vi "Multirecord Acquisition (FPGA).vi"() -> ()   [LabVIEW 2021]
doc: "Use this VI as a template for the reconfigurable oscilloscope acquisition design. The block diagram is divided into three main loops.\n\nRegister Bus: This loop initializes the registers that are needed to support the configuration of the device. The FIFO bus, on the left, allows all the other design libraries to communicate with one another. This loop is very important to support the proper behavior of the instrument design library components.\n\nAcquisition: Acquires data from the I/O channels and writes the data into the record memory using the <B>Write</B> VI of the Multirecord Acquisition instrument design library. This VI also evaluates the various acquisition triggers and decides whether to acquire each data value in record memory. The host level VI (Fetch Record.vi) can read acquired records from the DRAM. The data is stored in 2 DRAM banks, each with 768 MB of storage.\n\nFetch: The recorded data is retrieved when the <B>Fetch Single Record</B> VI is run from the host VI. The <B>Write to Fetch DMA FIFO</B> VI writes data to the acq.fetch fifo 0 to transmit record data form the FPGA to the record fetch VIs on the host. This DMA FIFO must have a predefined name based on the instance parameter. By default, it is 0 (since the associated terminal on the <B>Create Resources DRAM Write Read</B> VI is unwired), so the connected FIFO is named acq.fetch fifo 0."
uses:
  Trigger/SubVIs/Types/Trigger Type.ctl
  <instrlib>/_niInstr/Data Trigger/v1/Shared/Public/Level Configuration FXP(+-,18,1).ctl
  <instrlib>/_niInstr/Data Trigger/v1/Shared/Public/Level Configuration Trigger When.ctl
  <instrlib>/_niInstr/Data Trigger/v1/Shared/Public/Edge Configuration FXP(+-,18,1).ctl
  <instrlib>/_niInstr/Data Trigger/v1/Shared/Public/Edge Configuration Trigger Slope.ctl
  FPGA Interface Typedefinitions/Trigger Combination Type.ctl
  <vilib>/Platform/TimedLoop/XDataNode/timing_clust.ctl
  <vilib>/Platform/TimedLoop/XDataNode/nitl_modes.ctl
  <vilib>/Platform/TimedLoop/XDataNode/wakeup.ctl
  <instrlib>/_niInstr/FIFO Register Bus/v1/FPGA/niInstr FIFO Register Bus v1 FPGA.lvclass
  C:/Program Files (x86)/National Instruments/LabVIEW 2021/instr.lib/_niInstr/Instruction Framework/v1/FPGA/Interfaces/Instruction Producer/Instruction Producer.lvclass
  <instrlib>/_niInstr/Multirecord Acquisition/Common/v1/FPGA/niInstr Multirecord Acquisition Common v1 FPGA.lvclass
  C:/Program Files (x86)/National Instruments/LabVIEW 2021/instr.lib/_niInstr/Multirecord Acquisition/Interface/v1/FPGA/niInstr Multirecord Acquisition v1 FPGA.lvclass
  <vilib>/rvi/Emulation/niFpgaSctlEmulationGetInTimedLoop.vi
  <vilib>/rvi/Emulation/niFpgaEmulationReportErrorSimple.vi
  <vilib>/rvi/Emulation/niFpgaGetClockAttributes.vi
  <vilib>/rvi/Emulation/niFpgaCriticalErrorInLSC.vi
  <instrlib>/_niInstr/Multirecord Acquisition/Common/v1/FPGA/Private/Create Fetch DMA FIFO Resources U8x32.vi
  <instrlib>/_niInstr/Multirecord Acquisition/Common/v1/FPGA/Private/Create Resources DRAM U384x2 U768 Write Read.vi
  <vilib>/rvi/eio/common/nirviEmuTemplateMethod_errors.vi
  <instrlib>/HSAI-RIO/Config/Group A/v1/FPGA/Digital Correction/Validate 8 Channel Data.vi
  <instrlib>/HSAI-RIO/Config/Group A/v1/FPGA/Digital Correction/Digital Correction (8 Ch).vi
  <instrlib>/HSAI-RIO/Config/Group A/v1/FPGA/Digital Correction/FIR Filter (8 Ch).vi
  DSP/SubVIs/Integer decimationx8ch.vi
  Data Type Conversion/SubVIs/Remove Overflow FXP(+-,18,1)x8ch.vi
  <instrlib>/_niInstr/Channel/v1/FPGA/Private/Select/Select FXP(+-,18,1,)xNspcx8ch.vi
  Trigger/Trigger FXP(+,-,18,1).vi
  Data Type Conversion/SubVIs/Data Type Conversion FXP(+-,18,1) to I16x8ch.vi
  <instrlib>/_niInstr/Channel/v1/FPGA/Private/Select and Interleave/Select And Interleave I16xNspcx8ch.vi
  <instrlib>/_niInstr/Multirecord Acquisition/Interface/v1/FPGA/Private/Write I16 Wrapper.vi
  <vilib>/Platform/TimedLoop/XDataNode/XDataNode.xnode
  <vilib>/eio/EIONode/EIONode.xnode
  <instrlib>/_niInstr/Instruction Framework/v1/FPGA/Top Level Bus/Register Configuration/Register Configuration.lvclass
  <vilib>/Platform/TimedLoop/XDataNode/XDNodeRunTimeDep.lvlib
  <instrlib>/_niInstr/Multirecord Acquisition/Interface/v1/FPGA/niInstr Multirecord Acquisition v1 FPGA.lvclass
  <vilib>/rvi/LocalResourceManager/LocalResourceManager.xnode
  <vilib>/rvi/eio/common/nirviEmuReportErrorAndStop.vi
  <vilib>/rvi/DataTransferAndStorage/Container/Common/niFpgaContainerGetUniqueNameForEmu.vi
  <vilib>/rvi/DataTransferAndStorage/Container/Common/niFpgaContainerSetEmuInfo.vi
  <instrlib>/_niInstr/Channel/v1/FPGA/niInstr Channel v1 FPGA.lvlib
  <instrlib>/_niInstr/Basic Elements/v1/FPGA/niInstr Basic Elements v1 FPGA.lvlib
  <instrlib>/HSAI-RIO/Config/Group A/v1/FPGA/Digital Correction/Digital Correction.lvclass
  <instrlib>/HSAI-RIO/Config/Group A/v1/FPGA/Config Registers/Config Registers.lvclass
  <instrlib>/_niInstr/Data Trigger/v1/Shared/niInstr Data Trigger v1 Shared.lvlib
  Emulation/SubVIs/2 Element Generate Sine Cos Data FXP(+,-,14,1).vi
  <instrlib>/_niInstr/Multirecord Acquisition/Common/v1/FPGA/Private/Create Resources DRAM U384.vi
  <instrlib>/_niInstr/Multirecord Acquisition/Common/v1/FPGA/Private/Create Resources BRAM U384.vi
  <instrlib>/_niInstr/Multirecord Acquisition/Common/v1/FPGA/Private/Create Resources BRAM U768.vi
  C:/Program Files (x86)/National Instruments/LabVIEW 2021/instr.lib/_niInstr/Multirecord Acquisition/Common/v1/FPGA/niInstr Multirecord Acquisition Common v1 FPGA.lvclass
  FPGA Interface Typedefinitions/FPGA Interface Typedefinitions.lvlib
panel:
  in  "trigger.combination type":T1
  in  "trigger.rearm delay":u16=2
  in  "start trigger":bool=TRUE
  in  "trigger.type B":T2
  in  "reset":bool
  in  "trigger.edge B":T3
  in  "trigger.level B":T5
  in  "trigger.edge A":T3
  in  "trigger.level A":T5
  in  "trigger.type A":T2
  in  "trigger.channel A":u8
  in  "trigger.channel B":u8
  out "fifo reg bus data 0":u64
  out "fifo reg bus status 0":u32
  in  "fifo reg bus ctrl 0":u32
  out "overflow":bool
  in  "dsp.decimation factor":u16
  out "overload":bool
  in  "channel.enable mask":u16=65535 format="%.0b"
  in  "channel.number of channels":u8=8
  # "Register Bus Controls"
  # "FPGA"
  # "Acquisition Loop Controls"
  # "DSP"
  # "Trigger"
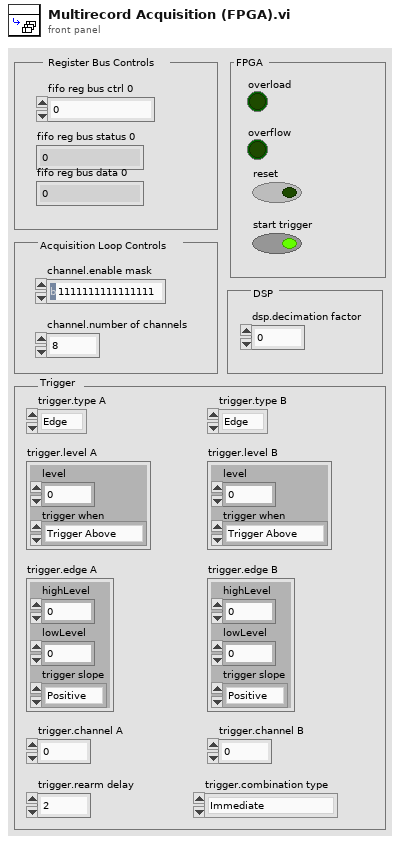
[diagram p1: front panel]
types:
  T1 = typedef "FPGA Interface Typedefinitions.lvlib/Trigger Combination Type.ctl" = enum16{"Immediate", "A", "B", "OR", "AND", "A THEN B", "B THEN A", "High Resolution"}
  T2 = typedef "Trigger Type.ctl" = enum16{"Edge", "Level", "Custom"}
  T3 = typedef "niInstr Data Trigger v1 Shared.lvlib/Edge Configuration FXP(+-,18,1).ctl" = cluster{"highLevel":fxp<+/-,18,1>, "lowLevel":fxp<+/-,18,1>, "trigger slope":T4}
  T4 = typedef "niInstr Data Trigger v1 Shared.lvlib/Edge Configuration Trigger Slope.ctl" = enum8{"Positive", "Negative"}
  T5 = typedef "niInstr Data Trigger v1 Shared.lvlib/Level Configuration FXP(+-,18,1).ctl" = cluster{"level":fxp<+/-,18,1>, "trigger when":T6}
  T6 = typedef "niInstr Data Trigger v1 Shared.lvlib/Level Configuration Trigger When.ctl" = enum8{"Trigger Above", "Trigger Below"}
  T7 = cluster{"memory 1":refnum<k21>, "memory 2":refnum<k21>}
  T8 = typedef "XDNodeRunTimeDep.lvlib/timing_clust.ctl" = cluster{"Expected End [f-1]":u64, "Actual End [f-1]":u64, "Finished Late? [f-1]":bool, "Expected End [i-1]":u64, "Actual End [i-1]":u64, "Finished Late? [i-1]":bool, "Expected Start [i]":u64, "Actual Start [i]":u64, "Expected Start [f]":u64, "Actual Start [f]":u64, "Source Name":string, "Structure Name":string, "Period":i64, "Deadline":i64, "Offset":i64, "Start":i64, "Priority":i32, "Timeout":i32, "Mode":T9, "Wakeup Reason":T10, "Error":errorcluster, "Source Type":string, "Secondary Source Type":string, "Global End Time":u64, "Global Start Time":u64, "Frame Duration":u64, "Iteration Duration":u64, "Assigned CPU":i32, "I/O Scan Engine Mode":u32}
  T9 = typedef "XDNodeRunTimeDep.lvlib/nitl_modes.ctl" = enum32{"No Change", "Process missed periods, maintain original phase", "Discard missed periods, maintain original phase", "Process missed periods, ignore original phase", "Discard missed periods, ignore original phase"}
  T10 = typedef "XDNodeRunTimeDep.lvlib/wakeup.ctl" = enum32{"Normal", "Aborted", "Asynchronous wakeup", "Timing source error", "Timed loop error", "Timeout"}
  T11 = cluster{"Channel 0":fxp<+/-,14,1>[], "Channel 1":fxp<+/-,14,1>[], "Channel 2":fxp<+/-,14,1>[], "Channel 3":fxp<+/-,14,1>[], "Channel 4":fxp<+/-,14,1>[], "Channel 5":fxp<+/-,14,1>[], "Channel 6":fxp<+/-,14,1>[], "Channel 7":fxp<+/-,14,1>[]}
  T12 = cluster{"Channel 0":fxp<+/-,18,1>[], "Channel 1":fxp<+/-,18,1>[], "Channel 2":fxp<+/-,18,1>[], "Channel 3":fxp<+/-,18,1>[], "Channel 4":fxp<+/-,18,1>[], "Channel 5":fxp<+/-,18,1>[], "Channel 6":fxp<+/-,18,1>[], "Channel 7":fxp<+/-,18,1>[]}
  T13 = cluster{"channel 0":fxp<+/-,18,1>[], "channel 1":fxp<+/-,18,1>[], "channel 2":fxp<+/-,18,1>[], "channel 3":fxp<+/-,18,1>[], "channel 4":fxp<+/-,18,1>[], "channel 5":fxp<+/-,18,1>[], "channel 6":fxp<+/-,18,1>[], "channel 7":fxp<+/-,18,1>[]}
  T14 = cluster{"channel 0":i16[], "channel 1":i16[], "channel 2":i16[], "channel 3":i16[], "channel 4":i16[], "channel 5":i16[], "channel 6":i16[], "channel 7":i16[]}
  T15 = typedef "niInstr Multirecord Acquisition v1 FPGA.lvclass/Timestamp.ctl" = cluster{"timestamp":u64, "valid":bool}
  T16 = typedef "niInstr Types v1 Shared.lvlib/Input Triggers.ctl" = cluster{"start":bool, "advance":bool, "reference":bool, "start trigger index":u16, "advance trigger index":u16, "reference trigger index":u16, "reference trigger correction cycle count":u32}
  T17 = typedef "niInstr Types v1 Shared.lvlib/Sample Format.ctl" = cluster{"bits per channel":u16, "samples per clock":u16, "channels":u8}
  T18 = typedef "niInstr Multirecord Acquisition v1 FPGA.lvclass/Events.ctl" = cluster{"ready for start":bool, "ready for advance":bool, "ready for reference":bool, "end of record":bool, "done":bool, "start trigger":bool, "advance trigger":bool, "reference trigger":bool, "start trigger index":u16, "advance trigger index":u16, "reference trigger index":u16}
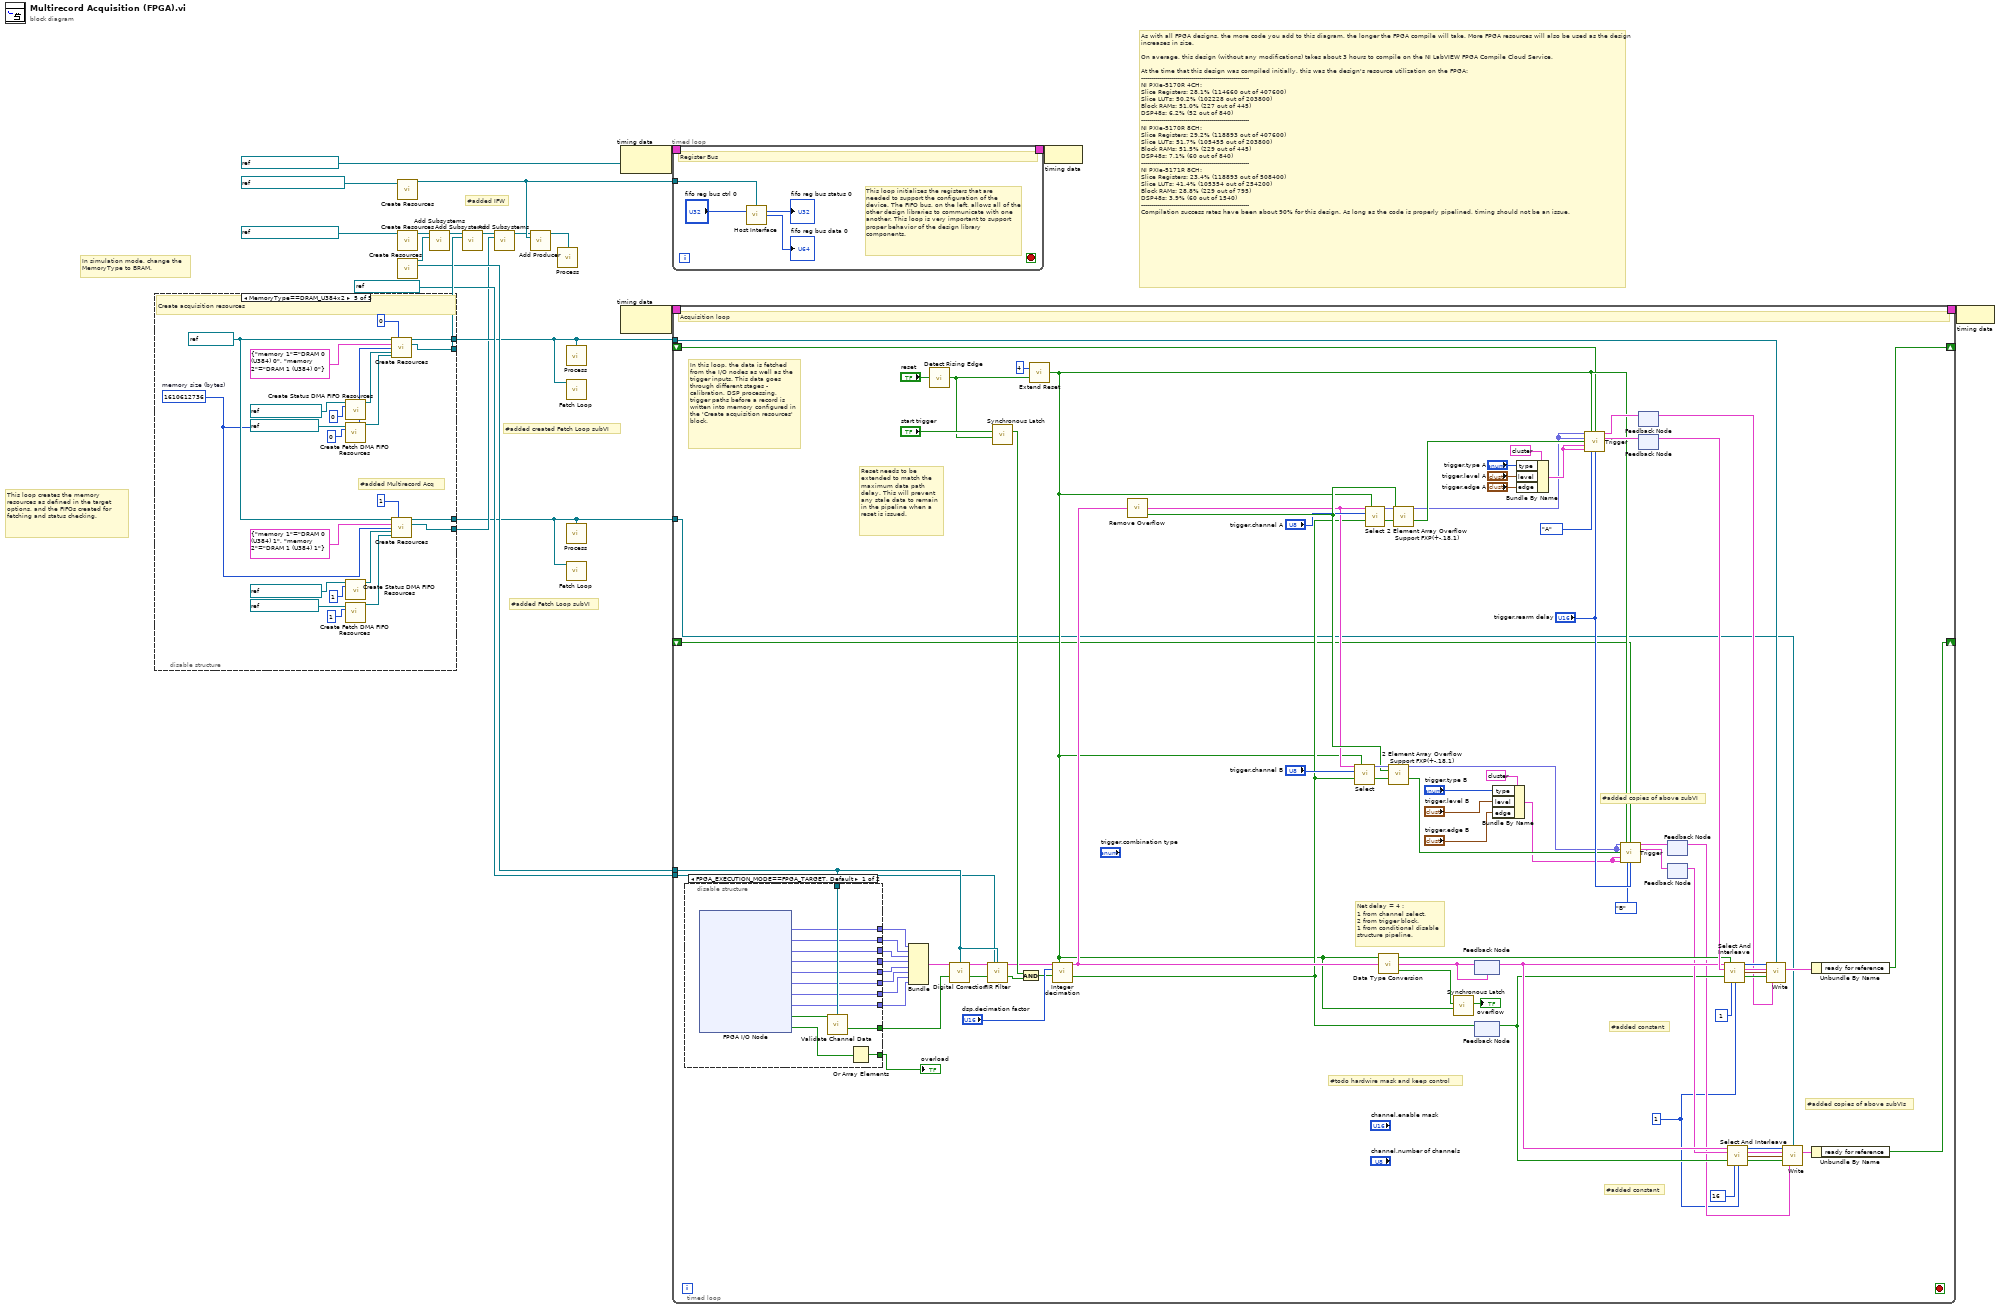
[diagram p0: block diagram]
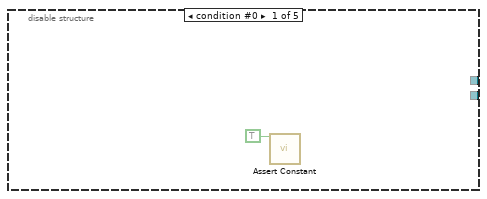
[diagram p2: hidden frame]
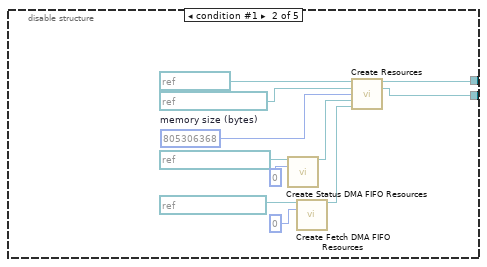
[diagram p3: hidden frame]
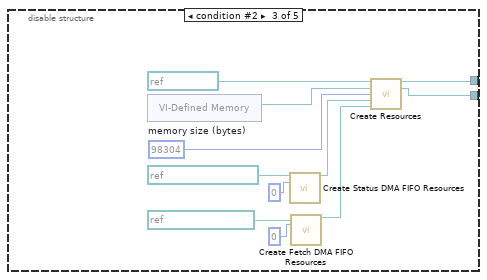
[diagram p4: hidden frame]
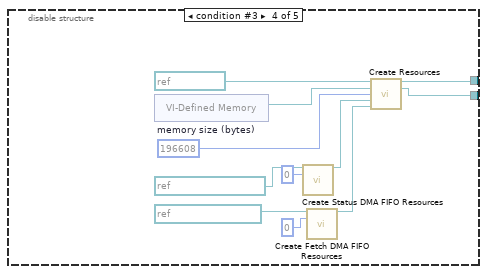
[diagram p5: hidden frame]
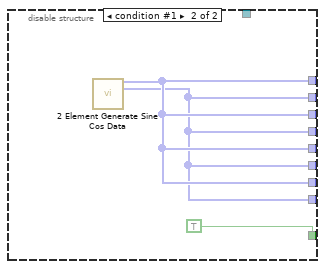
[diagram p6: hidden frame]
diagram:
  # "#added created Fetch Loop subVI"
  # "#added Fetch Loop subVI"
  # "#added IFW"
  # "In simulation mode, change the MemoryType to BRAM."
  # "This loop creates the memory resources as defined in the target options, and the FIFOs created for fetching and status checking."
  # "As with all FPGA designs, the more code you add to this diagram, the longer the FPGA compile will take. More FPGA resources will also be used as the design increases in size.\n\nOn average, this design (without any modifications) takes about 3 hours to compile on the NI LabVIEW FPGA Compile Cloud Service. \n\nAt the time that this design was compiled initially, this was the design's resource utilization on the FPGA:\n------------------------------------------------------\nNI PXIe-5170R 4CH:\nSlice Registers: 28.1% (114660 out of 407600)\nSlice LUTs: 50.2% (102228 out of 203800)\nBlock RAMs: 51.0% (227 out of 445)\nDSP48s: 6.2% (52 out of 840)\n------------------------------------------------------\nNI PXIe-5170R 8CH:\nSlice Registers: 29.2% (118893 out of 407600)\nSlice LUTs: 51.7% (105455 out of 203800)\nBlock RAMs: 51.5% (229 out of 445)\nDSP48s: 7.1% (60 out of 840)\n------------------------------------------------------\nNI PXIe-5171R 8CH:\nSlice Registers: 23.4% (118893 out of 508400)\nSlice LUTs: 41.4% (105354 out of 254200)\nBlock RAMs: 28.8% (229 out of 795)\nDSP48s: 3.9% (60 out of 1540)\n------------------------------------------------------\nCompilation success rates have been about 90% for this design. As long as the code is properly pipelined, timing should not be an issue."
  n1 = disable-structure shown="MemoryType==DRAM_U384x2" {
    disable-tunnel: [_ w30 w41 w52 w76] -> w3
    disable-tunnel: [_ w27 w37 w48 w73] -> w10
    disable-tunnel: [_ _ _ _ w56] -> w1
    disable-tunnel: [_ _ _ _ w55] -> w2
    frame condition #0 {
      n2 = call <instrlib>:"Assert Constant.vi"("constant terminal"=TRUE) -> ()  [unwired: 15 in]
    }
    frame condition #1 {
      w31 = u64 805306368  # memory size (bytes)
      n3 = call <instrlib>:"Create Status DMA FIFO Resources.vi"("status dma fifo in"=refnum<k21> "acq.status fifo 0" ("status dma fifo"), "fifo instance"=u8 0) -> ("status dma fifo out"=w22:refnum<class "niInstr Status FIFO v1 FPGA.lvclass">)  [unwired: 13 in]
      n4 = call-poly <instrlib>:"Create Fetch DMA FIFO Resources.vi"("fetch dma fifo in"=refnum<k21> "acq.fetch fifo 0", "fifo instance"=u8 0) -> ("fetch dma fifo out"=w28:refnum<class "niInstr Fetch FIFO v1 FPGA.lvclass">)  [unwired: 13 in]
      n5 = call-poly <instrlib>:"Create Resources.vi"("memory clock"=refnum<k21> "160MHz" ("process clock"), "memory"=refnum<k21> "DRAM 0 (U384)" ("dram"), "memory size (bytes)"=w31, "status dma fifo resources"=w22, "fetch dma fifo resources"=w28) -> ("acquisition resources"=w30:refnum<class "niInstr Multirecord Acquisition Common v1 FPGA.lvclass">, "acquisition subsystem"=w27:refnum<class "Address Space Collection.lvclass">)  [unwired: 9 in]
    }
    frame condition #2 {
      w42 = u64 98304  # memory size (bytes)
      n6 = xnode "VI-Defined Memory"() -> ("Memory Out"=w43:refnum<k21>)
      n7 = call <instrlib>:"Create Status DMA FIFO Resources.vi"("status dma fifo in"=refnum<k21> "acq.status fifo 0" ("status dma fifo"), "fifo instance"=u8 0) -> ("status dma fifo out"=w34:refnum<class "niInstr Status FIFO v1 FPGA.lvclass">)  [unwired: 13 in]
      n8 = call-poly <instrlib>:"Create Fetch DMA FIFO Resources.vi"("fetch dma fifo in"=refnum<k21> "acq.fetch fifo 0", "fifo instance"=u8 0) -> ("fetch dma fifo out"=w38:refnum<class "niInstr Fetch FIFO v1 FPGA.lvclass">)  [unwired: 13 in]
      n9 = call-poly <instrlib>:"Create Resources.vi"("memory clock"=refnum<k21> "160MHz" ("process clock"), "memory"=w43, "memory size (bytes)"=w42, "status dma fifo resources"=w34, "fetch dma fifo resources"=w38) -> ("acquisition resources"=w41:refnum<class "niInstr Multirecord Acquisition Common v1 FPGA.lvclass">, "acquisition subsystem"=w37:refnum<class "Address Space Collection.lvclass">)  [unwired: 9 in]
    }
    frame condition #3 {
      w53 = u64 196608  # memory size (bytes)
      n10 = xnode "VI-Defined Memory"() -> ("Memory Out"=w54:refnum<k21>)
      n11 = call <instrlib>:"Create Status DMA FIFO Resources.vi"("status dma fifo in"=refnum<k21> "acq.status fifo 0" ("status dma fifo"), "fifo instance"=u8 0) -> ("status dma fifo out"=w46:refnum<class "niInstr Status FIFO v1 FPGA.lvclass">)  [unwired: 13 in]
      n12 = call-poly <instrlib>:"Create Fetch DMA FIFO Resources.vi"("fetch dma fifo in"=refnum<k21> "acq.fetch fifo 0", "fifo instance"=u8 0) -> ("fetch dma fifo out"=w49:refnum<class "niInstr Fetch FIFO v1 FPGA.lvclass">)  [unwired: 13 in]
      n13 = call-poly <instrlib>:"Create Resources.vi"("memory clock"=refnum<k21> "160MHz" ("process clock"), "memory"=w54, "memory size (bytes)"=w53, "status dma fifo resources"=w46, "fetch dma fifo resources"=w49) -> ("acquisition resources"=w52:refnum<class "niInstr Multirecord Acquisition Common v1 FPGA.lvclass">, "acquisition subsystem"=w48:refnum<class "Address Space Collection.lvclass">)  [unwired: 9 in]
    }
    frame condition #4 (active) {
      w60 = refnum<k21> "160MHz" ("process clock")
      w57 = u64 1610612736  # memory size (bytes)
      # "#added Multirecord Acq"
      # "Create acquisition resources"
      n14 = call-poly <instrlib>:"Create Fetch DMA FIFO Resources.vi"("fetch dma fifo in"=refnum<k21> "acq.fetch fifo 0", "fifo instance"=u8 0) -> ("fetch dma fifo out"=w75:refnum<class "niInstr Fetch FIFO v1 FPGA.lvclass">)  [unwired: 13 in]
      n15 = call-poly <instrlib>:"Create Fetch DMA FIFO Resources.vi"("fetch dma fifo in"=refnum<k21> "acq.fetch fifo 1", "fifo instance"=u8 1) -> ("fetch dma fifo out"=w61:refnum<class "niInstr Fetch FIFO v1 FPGA.lvclass">)  [unwired: 13 in]
      n16 = call <instrlib>:"Create Status DMA FIFO Resources.vi"("status dma fifo in"=refnum<k21> "acq.status fifo 0" ("status dma fifo"), "fifo instance"=u8 0) -> ("status dma fifo out"=w70:refnum<class "niInstr Status FIFO v1 FPGA.lvclass">)  [unwired: 13 in]
      n17 = call <instrlib>:"Create Status DMA FIFO Resources.vi"("status dma fifo in"=refnum<k21> "acq.status fifo 1" ("status dma fifo"), "fifo instance"=u8 1) -> ("status dma fifo out"=w65:refnum<class "niInstr Status FIFO v1 FPGA.lvclass">)  [unwired: 13 in]
      n18 = call-poly <instrlib>:"Create Resources.vi"("memory clock"=w60, "instance"=u8 0, "memory"=T7 {"memory 1"="DRAM 0 (U384) 0", "memory 2"="DRAM 1 (U384) 0"}, "memory size (bytes)"=w57, "status dma fifo resources"=w70, "fetch dma fifo resources"=w75) -> ("acquisition resources"=w76:refnum<class "niInstr Multirecord Acquisition Common v1 FPGA.lvclass">, "acquisition subsystem"=w73:refnum<class "Address Space Collection.lvclass">)  [unwired: 8 in]
      n19 = call-poly <instrlib>:"Create Resources.vi"("memory clock"=w60, "instance"=u8 1, "memory"=T7 {"memory 1"="DRAM 0 (U384) 1", "memory 2"="DRAM 1 (U384) 1"}, "memory size (bytes)"=w57, "status dma fifo resources"=w65, "fetch dma fifo resources"=w61) -> ("acquisition resources"=w56:refnum<class "niInstr Multirecord Acquisition Common v1 FPGA.lvclass">, "acquisition subsystem"=w55:refnum<class "Address Space Collection.lvclass">)  [unwired: 8 in]
    }
  }
  n20 = call <instrlib>:"Create Resources.vi"("instruction fifo"=refnum<k21> "reg.host instruction fifo 0" ("FIFO")) -> ("fifo register bus"=w9:refnum<class "niInstr FIFO Register Bus v1 FPGA.lvclass">)  [unwired: 14 in]
  n21 = call <instrlib>:"Create Resources.vi"("register clock"=refnum<k21> "40 MHz Onboard Clock" ("Source Name")) -> ("register configuration"=w13:refnum<class "Register Configuration.lvclass">)  [unwired: 14 in]
  n22 = call <instrlib>:"Create Resources.vi"() -> ("config subsystems"=w11:refnum<class "Address Space Collection.lvclass">, "digital correction resources"=w6:refnum<class "Digital Correction.lvclass">)  [unwired: 14 in]
  n23 = call-dynamic "Add Subsystems.vi"("register configuration in"=w13, "subsystems"=w11) -> ("register configuration out"=w12:refnum<class "Register Configuration.lvclass">)  [unwired: 13 in]
  n24 = call-dynamic "Add Subsystems.vi"("register configuration in"=w12, "subsystems"=w10) -> ("register configuration out"=w5:refnum<class "Register Configuration.lvclass">)  [unwired: 13 in]
  n25 = call-dynamic "Add Subsystems.vi"("register configuration in"=w5, "subsystems"=w2) -> ("register configuration out"=w4:refnum<class "Register Configuration.lvclass">)  [unwired: 13 in]
  n26 = call-dynamic "Add Producer.vi"("register configuration in"=w4, "instruction producer"=w9) -> ("register configuration out"=w8:refnum<class "Register Configuration.lvclass">)  [unwired: 13 in]
  n27 = call-dynamic "Process.vi"("register configuration"=w8) -> ()  [unwired: 15 in]
  n28 = call-dynamic "Process.vi"("acquisition resources"=w3) -> ()  [unwired: 15 in]
  n29 = call "Fetch Loop.vi"("niInstr Multirecord Acquisition Common v1 FPGA in"=w3) -> ()  [unwired: 11 in]
  n30 = call-dynamic "Process.vi"("acquisition resources"=w1) -> ()  [unwired: 15 in]
  n31 = call "Fetch Loop.vi"("niInstr Multirecord Acquisition Common v1 FPGA in"=w1) -> ()  [unwired: 11 in]
  n32 = node-c288(refnum<k21> "40 MHz Onboard Clock" ("Source Name")) -> (w20:T8)
  n33 = node-c288() -> (w18:T8)  [unwired: 1 in]
  n34 = timed-loop {
    timing: w20 -> [_]
    timing-out: [_] -> w19
    tunnel: w9 -> [w80]
    stop <- _ stop-if-true
    # "This loop initializes the registers that are needed to support the configuration of the device. The FIFO bus, on the left, allows all of the other design libraries to communicate with one another. This loop is very important to support proper behavior of the design library components."
    # "Register Bus"
    n35 = call <instrlib>:"Host Interface.vi"("fifo register bus"=w80, "fifo reg bus ctrl 0"="fifo reg bus ctrl 0") -> ("fifo reg bus status 0"=→"fifo reg bus status 0":u32, "fifo reg bus data 0"=→"fifo reg bus data 0":u64)  [unwired: 12 in]
  }
  n36 = timed-loop {
    timing: w18 -> [_]
    timing-out: [_] -> w17
    tunnel: w3 -> [w131]
    tunnel: w6 -> [w135]
    shift-right: [w157] -> _
    shift-left: _ -> [w109]
    tunnel: refnum<k21> "Data Clock x2" -> [w132]
    tunnel: w1 -> [w93]
    shift-right: [w101] -> _
    shift-left: _ -> [w100]
    stop <- _ stop-if-true
    w85 = u8 1 ("number of channels to interleave")
    # "#added constant"
    # "#added constant"
    # "#todo hardwire mask and keep control"
    # "#added copies of above subVI"
    # "#added copies of above subVIs"
    # "Net delay = 4 :\n1 from channel select.\n2 from trigger block.\n1 from conditional disable structure pipeline."
    # "Reset needs to be extended to match the maximum data path delay. This will prevent any stale data to remain in the pipeline when a reset is issued."
    # "In this loop, the data is fetched from the I/O nodes as well as the trigger inputs. This data goes through different stages - calibration, DSP processing, trigger paths before a record is written into memory configured in the 'Create acquisition resources' block."
    # "Acquisition loop"
    n37 = disable-structure shown="FPGA_EXECUTION_MODE==FPGA_TARGET, Default" {
      disable-tunnel: [w175 w180] -> w130
      disable-tunnel: [w174 w179] -> w129
      disable-tunnel: [w173 w180] -> w128
      disable-tunnel: [w172 w179] -> w127
      disable-tunnel: [w171 w180] -> w126
      disable-tunnel: [w170 w179] -> w125
      disable-tunnel: [w169 w180] -> w123
      disable-tunnel: [w168 w179] -> w124
      disable-tunnel: [w165 TRUE ("ADC Data Valid")] -> w121
      disable-tunnel: w135 -> [w176 _]
      disable-tunnel: [w166 _] -> w164
      frame condition #0 (active) {
        # "I/O Nodes"
        n38 = xnode "FPGA I/O Node"() -> ("Channel 0"=w175:fxp<+/-,14,1>[], "Channel 1"=w174:fxp<+/-,14,1>[], "Channel 2"=w173:fxp<+/-,14,1>[], "Channel 3"=w172:fxp<+/-,14,1>[], "Channel 4"=w171:fxp<+/-,14,1>[], "Channel 5"=w170:fxp<+/-,14,1>[], "Channel 6"=w169:fxp<+/-,14,1>[], "Channel 7"=w168:fxp<+/-,14,1>[], "Channel Data Valid"=w177:bool[], "Channel Overload"=w167:bool[])  [unwired: 10 in, 10 out]
        n39 = call-poly <instrlib>:"Validate Channel Data.vi"("channel data valid"=w177, "digital correction resources"=w176) -> ("expected data valid"=w165:bool)  [unwired: 13 in]
        n40 = Or Array Elements(Boolean array=w167) -> (logical OR=w166:bool)
      }
      frame condition #1 {
        n41 = call-poly "2 Element Generate Sine Cos Data.vi"() -> ("sine data"=w180:fxp<+/-,14,1>[], "cosine data"=w179:fxp<+/-,14,1>[])  [unwired: 14 in]
      }
    }
    "overload" <- w164
    n42 = Bundle("Channel 0"=w130, "Channel 1"=w129, "Channel 2"=w128, "Channel 3"=w127, "Channel 4"=w126, "Channel 5"=w125, "Channel 6"=w123, "Channel 7"=w124) -> (w122:T11)  [unwired: 1 in]
    n43 = call <instrlib>:"Detect Rising Edge.vi"("signal"="reset") -> ("edge detected"=w134:bool)  [unwired: 14 in]
    n44 = call-poly <instrlib>:"Digital Correction.vi"("channel data in"=w122, "digital correction resources"=w135, "input valid"=w121) -> ("corrected channel data out"=w115:T12, "output valid"=w114:bool)  [unwired: 11 in]
    n45 = call-poly <instrlib>:"FIR Filter.vi"("data in"=w115, "data clock x2"=w132, "digital correction resources"=w135, "input valid"=w114) -> ("data out"=w112:T12, "output valid"=w113:bool)  [unwired: 9 in, 1 out]
    n46 = call <instrlib>:"Synchronous Latch.vi"("clear"=w134, "set"="start trigger") -> ("out"=w143:bool)  [unwired: 9 in]
    n47 = And(x=w143, y=w113) -> (x .and. y?=w116:bool)
    n48 = call "Extend Reset.vi"("reset in"=w134, "number of cycles"=u8 4) -> ("reset out"=w110:bool)
    n49 = call-poly "Integer decimation.vi"("data in"=w112, "reset"=w110, "decimation factor"="dsp.decimation factor", "input valid"=w116) -> ("data out"=w118:T13, "output valid"=w117:bool)  [unwired: 9 in, 1 out]
    n50 = call-poly "Remove Overflow.vi"("data in"=w118) -> ("overflow"=w145:bool, "data out"=w119:T13)  [unwired: 3 in]
    n51 = call-poly <instrlib>:"Select.vi"("data in"=w119, "reset"=w110, "channel index"="trigger.channel B", "input valid"=w117) -> ("channel out"=w146:fxp<+/-,18,1>[], "output valid"=w91:bool)  [unwired: 10 in]
    n52 = call-poly <instrlib>:"Select.vi"("data in"=w119, "reset"=w110, "channel index"="trigger.channel A", "input valid"=w117) -> ("channel out"=w147:fxp<+/-,18,1>[], "output valid"=w92:bool)  [unwired: 10 in]
    n53 = call-poly "Data Type Conversion.vi"("data in"=w118) -> ("overflow"=w120:bool, "data out"=w111:T14)  [unwired: 3 in]
    n54 = call "2 Element Array Overflow Support FXP(+-,18,1).vi"("data in"=w146, "overflow"=w145) -> ("data out"=w86:fxp<+/-,18,1>[])  [unwired: 13 in]
    n55 = call "2 Element Array Overflow Support FXP(+-,18,1).vi"("data in"=w147, "overflow"=w145) -> ("data out"=w87:fxp<+/-,18,1>[])  [unwired: 13 in]
    n56 = call <instrlib>:"Synchronous Latch.vi"("clear"=w110, "set"=w120) -> ("out"=→"overflow":bool)  [unwired: 9 in]
    n57 = feedback #1(w111) -> (w99:T14)
    n58 = feedback-in #1(w111) -> ()
    n59 = feedback #2() -> (w95:bool)  [unwired: 1 in]
    n60 = feedback-in #2(w117) -> ()
    n61 = Bundle By Name(cluster=cluster{"type":T2, "level":T5, "edge":T3} {"type"=enum."Edge", "level"={"level"=0.0, "trigger when"=enum."Trigger Above"}, "edge"={"highLevel"=0.0, "lowLevel"=0.0, "trigger slope"=enum."Positive"}} ("trigger.A"), "type"="trigger.type B", "level"="trigger.level B", "edge"="trigger.edge B") -> (w88:cluster{"type":T2, "level":T5, "edge":T3})
    n62 = Bundle By Name(cluster=cluster{"type":T2, "level":T5, "edge":T3} {"type"=enum."Edge", "level"={"level"=0.0, "trigger when"=enum."Trigger Above"}, "edge"={"highLevel"=0.0, "lowLevel"=0.0, "trigger slope"=enum."Positive"}} ("trigger.A"), "type"="trigger.type A", "level"="trigger.level A", "edge"="trigger.edge A") -> (w89:cluster{"type":T2, "level":T5, "edge":T3})
    n63 = call-poly "Trigger.vi"("data A"=w87, "reset"=w110, "trigger.ready for reference"=w109, "data B"=w87, "input valid"=w92, "trigger.A"=w89, "trigger.B"=w89, "trigger.combination type"=Trigger_Combination_Type."A" ("trigger.combination type A"), "rearm delay"="trigger.rearm delay") -> ("timestamps"=w140:T15, "trigger.out"=w142:T16)  [unwired: 4 in, 1 out]
    n64 = call-poly "Trigger.vi"("data A"=w86, "reset"=w110, "trigger.ready for reference"=w100, "data B"=w86, "input valid"=w91, "trigger.A"=w88, "trigger.B"=w88, "trigger.combination type"=Trigger_Combination_Type."B" ("trigger.combination type B"), "rearm delay"="trigger.rearm delay") -> ("timestamps"=w98:T15, "trigger.out"=w97:T16)  [unwired: 4 in, 1 out]
    n65 = feedback #3() -> (w139:T15)  [unwired: 1 in]
    n66 = feedback-in #3(w140) -> ()
    n67 = feedback #4() -> (w141:T16)  [unwired: 1 in]
    n68 = feedback-in #4(w142) -> ()
    n69 = feedback #5() -> (w94:T15)  [unwired: 1 in]
    n70 = feedback-in #5(w98) -> ()
    n71 = feedback #6() -> (w96:T16)  [unwired: 1 in]
    n72 = feedback-in #6(w97) -> ()
    n73 = call-poly <instrlib>:"Select And Interleave.vi"("data in"=w99, "reset"=w110, "triggers in"=w141, "input valid"=w95, "channel enable mask"=u16 1 ("channel.enable mask"), "number of channels to interleave"=w85) -> ("interleaved data out"=w163:i16[], "triggers out"=w162:T16, "sample format out"=w161:T17, "output valid"=w160:bool)  [unwired: 5 in, 1 out]
    n74 = call-poly <instrlib>:"Select And Interleave.vi"("data in"=w99, "triggers in"=w96, "input valid"=w95, "channel enable mask"=u16 16 ("channel.enable mask"), "number of channels to interleave"=w85) -> ("interleaved data out"=w102:i16[], "triggers out"=w103:T16, "sample format out"=w104:T17, "output valid"=w105:bool)  [unwired: 6 in, 1 out]
    n75 = call-poly <instrlib>:"Write.vi"("data"=w163, "acquisition resources"=w131, "triggers"=w162, "sample format"=w161, "data valid"=w160, "timestamp"=w139) -> ("events"=w158:T18)  [unwired: 7 in, 2 out]
    n76 = call-poly <instrlib>:"Write.vi"("data"=w102, "acquisition resources"=w93, "triggers"=w103, "sample format"=w104, "data valid"=w105, "timestamp"=w94) -> ("events"=w106:T18)  [unwired: 7 in, 2 out]
    n77 = Unbundle By Name(w158) -> ("ready for reference"=w157:bool)
    n78 = Unbundle By Name(w106) -> ("ready for reference"=w101:bool)
  }
  n79 = node-c288(w19) -> ()
  n80 = node-c288(w17) -> ()
